vi "方格图标定.vi"() -> ()   [LabVIEW 2018]
uses:
  <vilib>/vision/Calibration.llb/Calibration Reference Points.ctl
  <vilib>/vision/Calibration.llb/Distortion Model.ctl
  <vilib>/vision/Calibration.llb/Distortion Model Types.ctl
  <vilib>/Utility/error.llb/DialogType.ctl
  <vilib>/vision/NI_Vision_Development_Module.lvlib
panel:
  in  "布尔":bool
  out "ROI Descriptor":T1 {"Contours"."Type" items=["No Selection", "Point", "Line", "Rectangle", "Oval", "Polygon", "Freehand Region", "Annulus", "Unused2", "Unused3", "Broken Line", "Freehand Line", "Rotated Rectangle"]}
  in  "生成均值坐标点":bool
  in  "角点增加":bool
  in  "停止按钮":bool
  in  "进行图像标定":bool
  out "标定完成":bool
  out "Location":cluster{"X":sgl, "Y":sgl}
  in  "X轴方向间距":i32
  in  "Y轴方向间距":i32
  in  "Reference Points":T2
  in  "单位选择":u16(ring) items=["Undefined", "Angstr", "Micrometer", "Millimeter", "Centimeter", "Meter", "Kilometer", "Microinch", "Inch", "Feet", "Nautical miles", "Standardmiles", "Steps"]
  out "角点图":T4(plugin-control)
  out "图像尺寸":cluster{"X":u32, "Y":u32}
  in  "删除按钮":bool
  in  "角点检测参数设置":T5={"角点检测算法选择"=0, "Kernel 尺寸"=3, "最小的角点强度"=20.0} {"角点检测算法选择" items=["Harris Corner", "Shi-Tomasi Corner"]; "Kernel 尺寸" min=3 max=7 step=2}
  in  "刷新按钮":bool
  # "方格图标定"
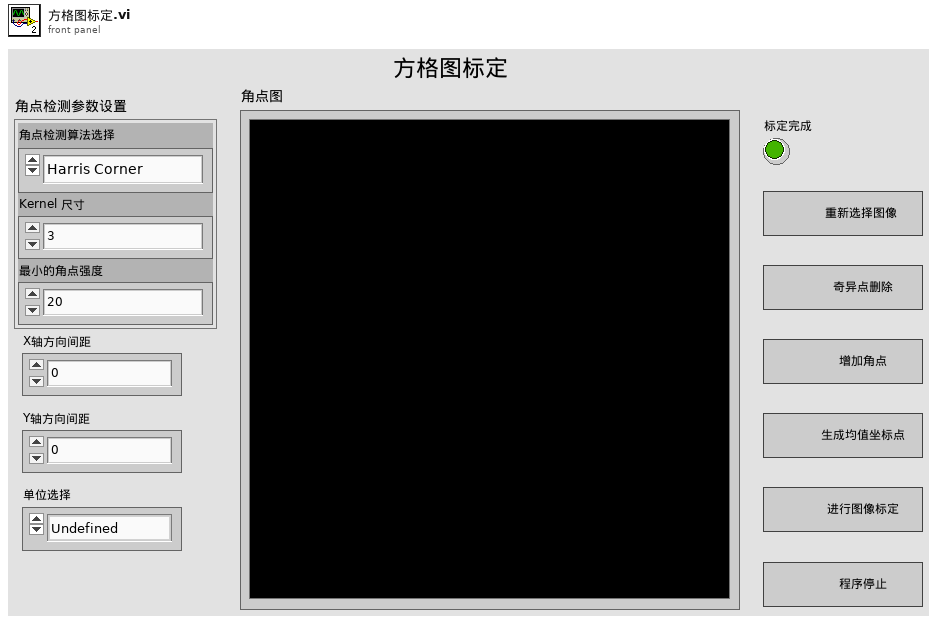
[diagram p1: front panel]
types:
  T1 = typedef "ROI Descriptor" = cluster{"Global Rectangle":i32[], "Contours":cluster{"ID":enum32{"External", "Internal"}, "Type":u32, "Coordinates":i32[]}[]}
  T2 = typedef "Calibration Reference Points.ctl" = cluster{"Pixel Coordinates":cluster{"X":dbl, "Y":dbl}[], "Real World Coordinates":cluster{"X":dbl, "Y":dbl}[], "Unit":T3, "Image Size":cluster{"X":u32, "Y":u32}}
  T3 = typedef "Image Unit" = enum32{"Undefined", "Angström", "Micrometer", "Millimeter", "Centimeter", "Meter", "Kilometer", "Microinch", "Inch", "Feet", "Nautical miles", "Standard miles", "Steps"}
  T4 = typedef "IMAQ Image.ctl" = refnum<image>
  T5 = cluster{"角点检测算法选择":u16, "Kernel 尺寸":i32, "最小的角点强度":dbl}
  T6 = enum8{"Enabled", "Disabled", "Disabled and Grayed Out"}
  T7 = typedef "Image Type" = u32
  T8 = typedef "IMAQ Rectangle" = cluster{"Left":i32, "Top":i32, "Right":i32, "Bottom":i32, "Rotation":dbl}
  T9 = enum32{"Invalid", "Standard", "Closed", "Hidden", "Minimized", "Maximized"}
  T10 = typedef "DialogType.ctl" = u16
  T11 = typedef "Distortion Model.ctl" = cluster{"Distortion Model":T12, "Polynomial Model Setup":cluster{"Radial Coefficient":u32, "Tangential Coefficients ":bool}}
  T12 = typedef "Distortion Model Types.ctl" = i32
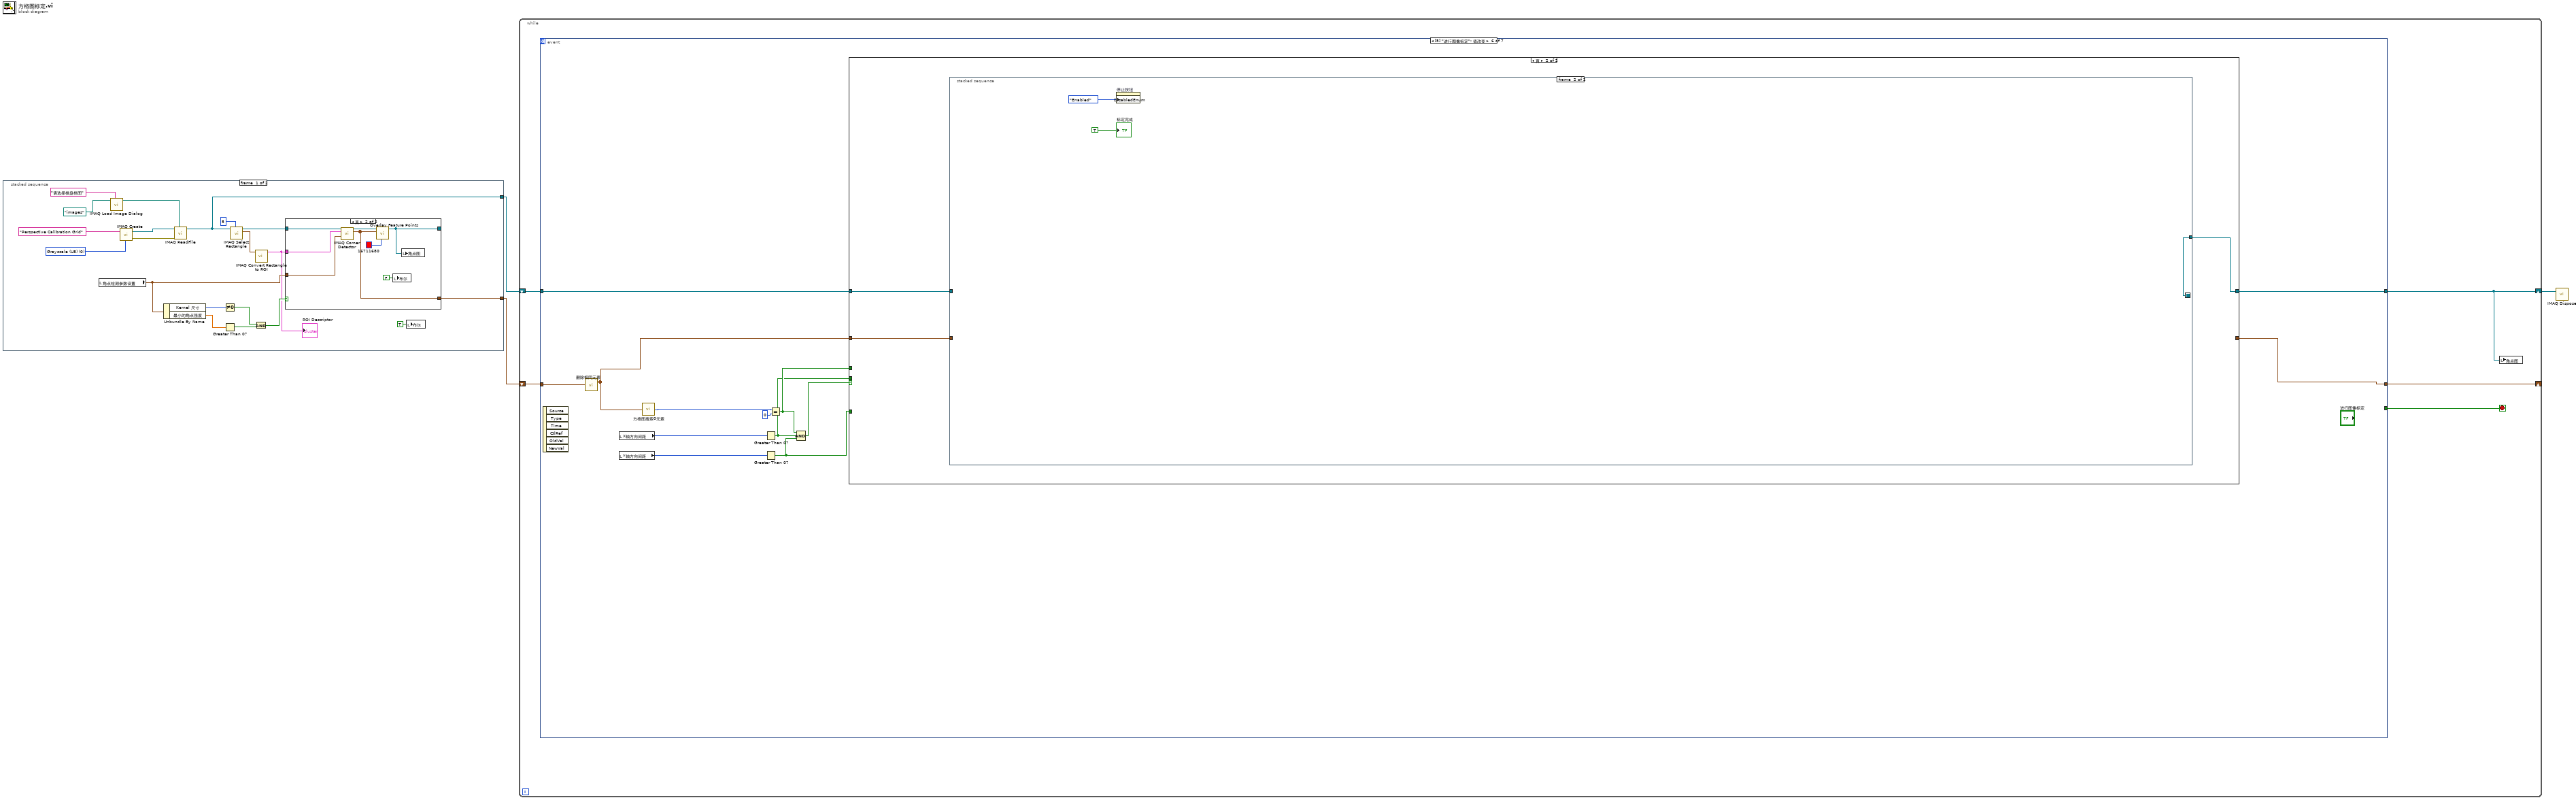
[diagram p0: block diagram]
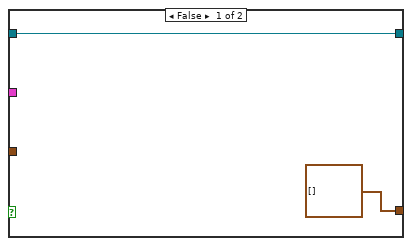
[diagram p2: hidden frame]
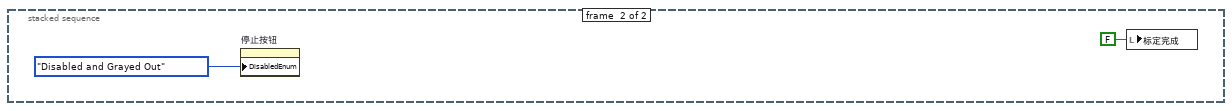
[diagram p3: hidden frame]
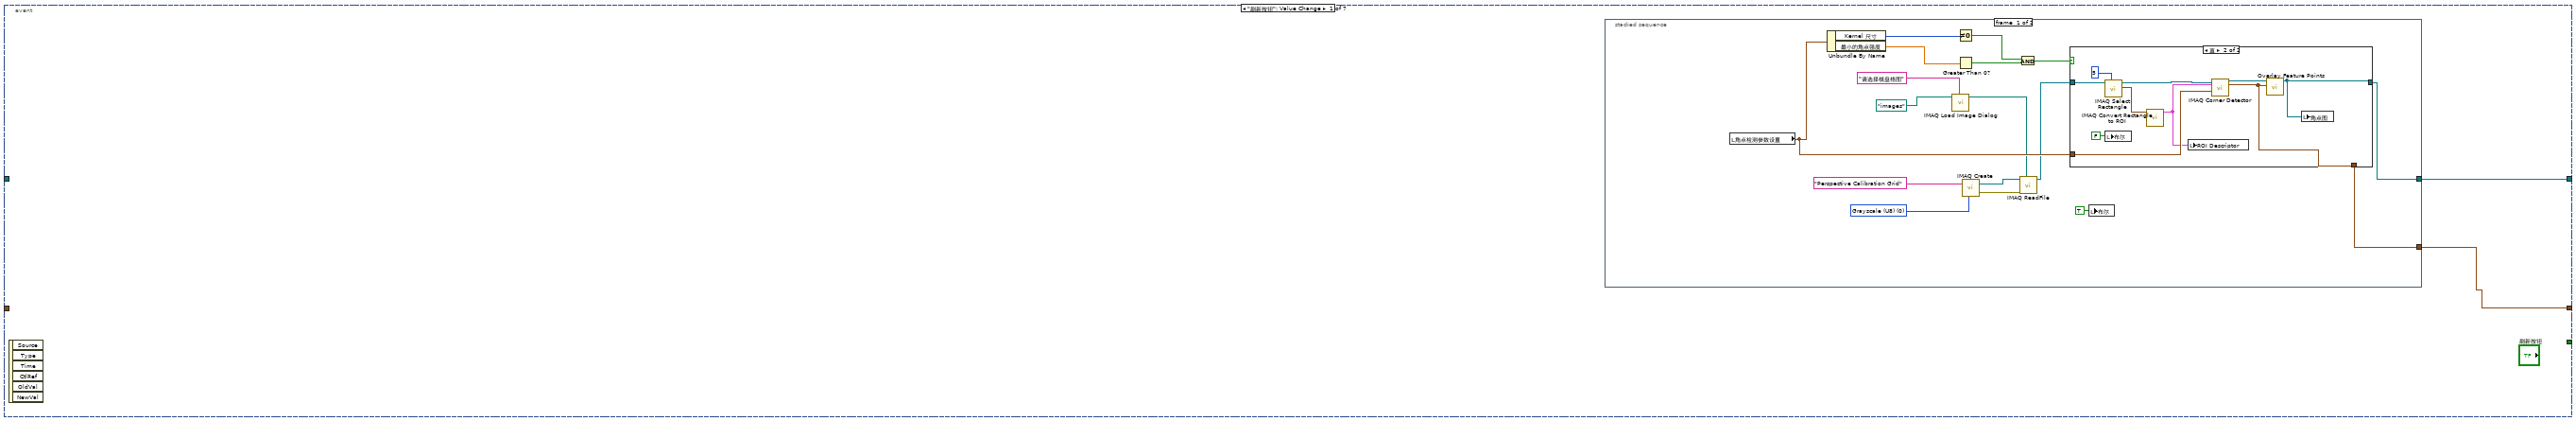
[diagram p4: hidden frame]
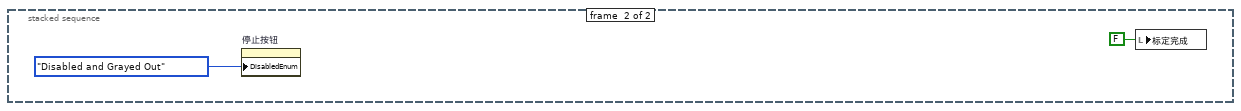
[diagram p6: hidden frame]
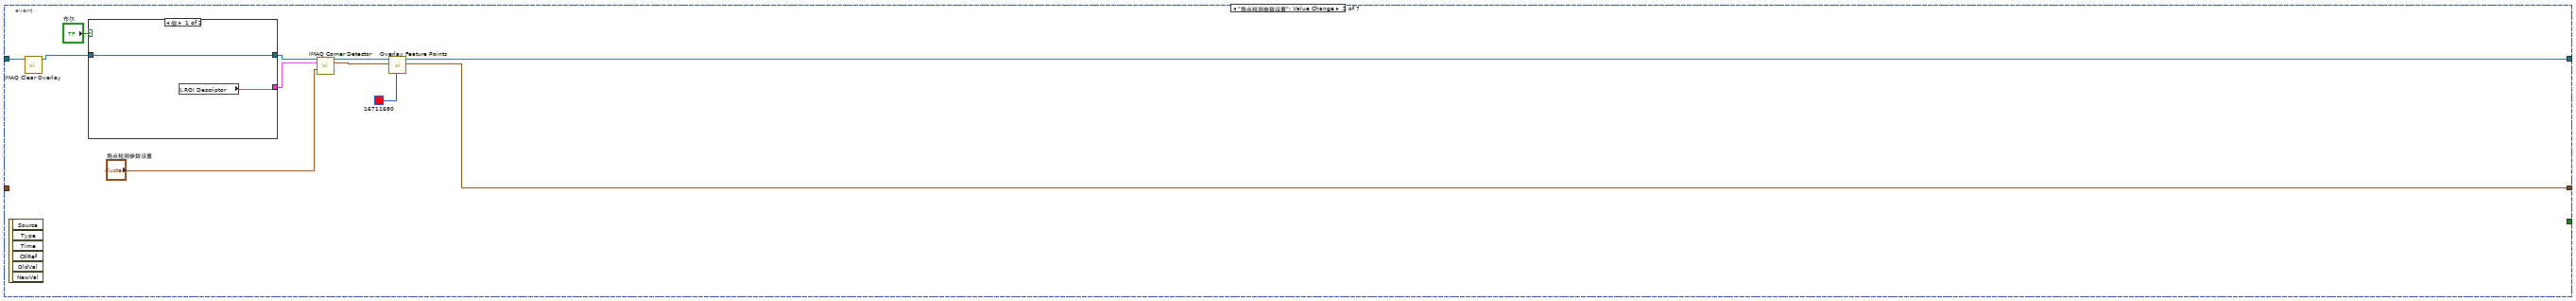
[diagram p7: hidden frame]
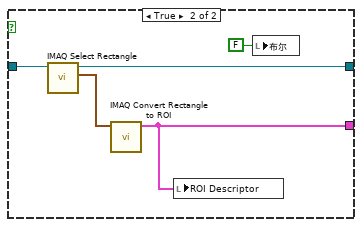
[diagram p8: hidden frame]
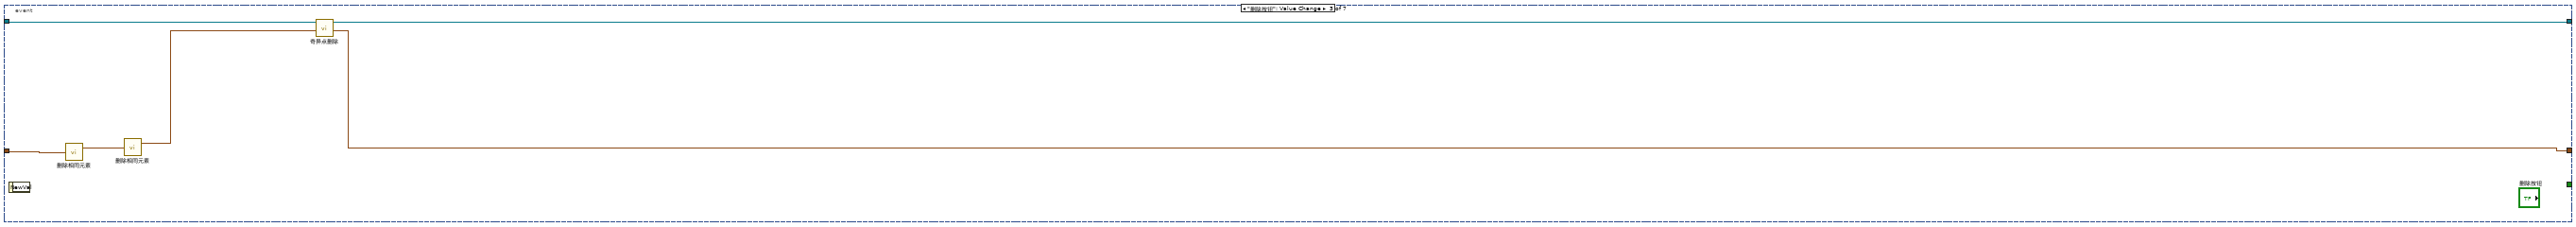
[diagram p9: hidden frame]
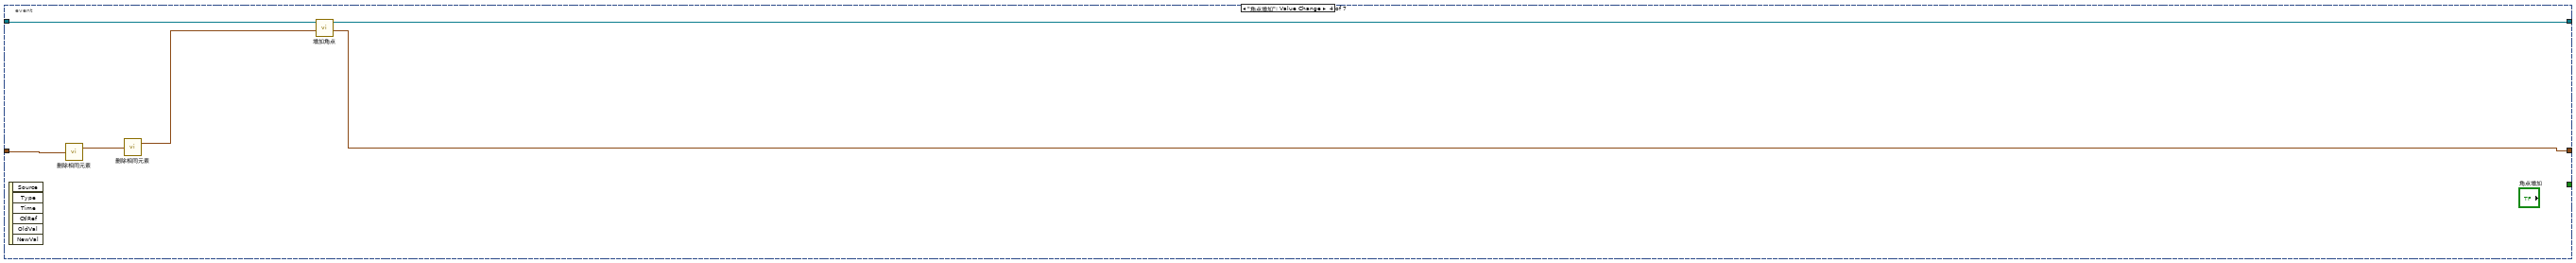
[diagram p10: hidden frame]
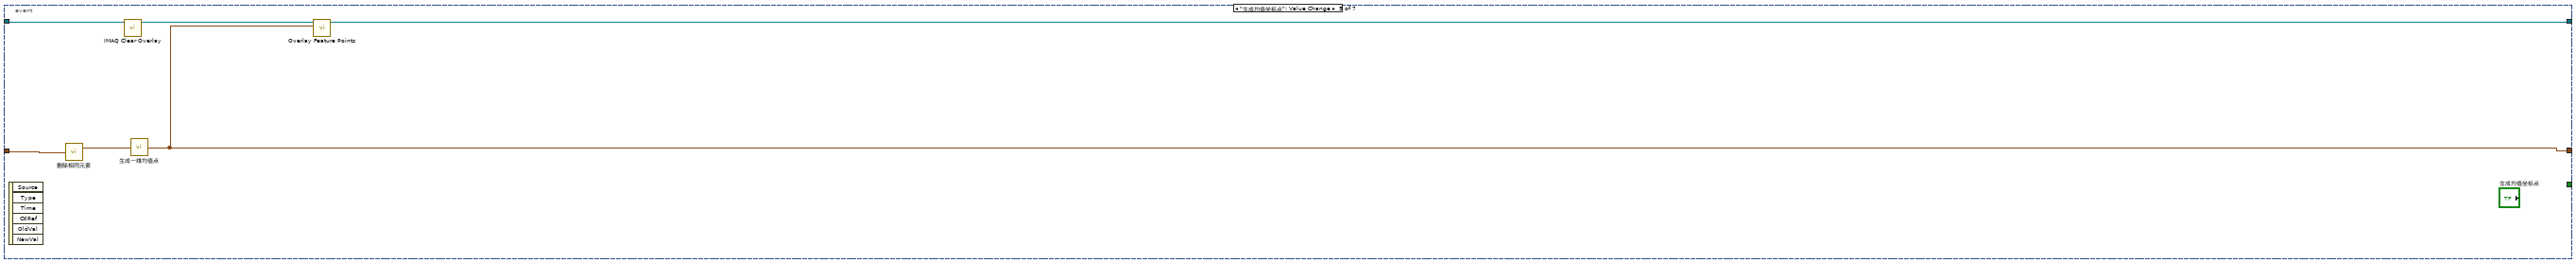
[diagram p11: hidden frame]
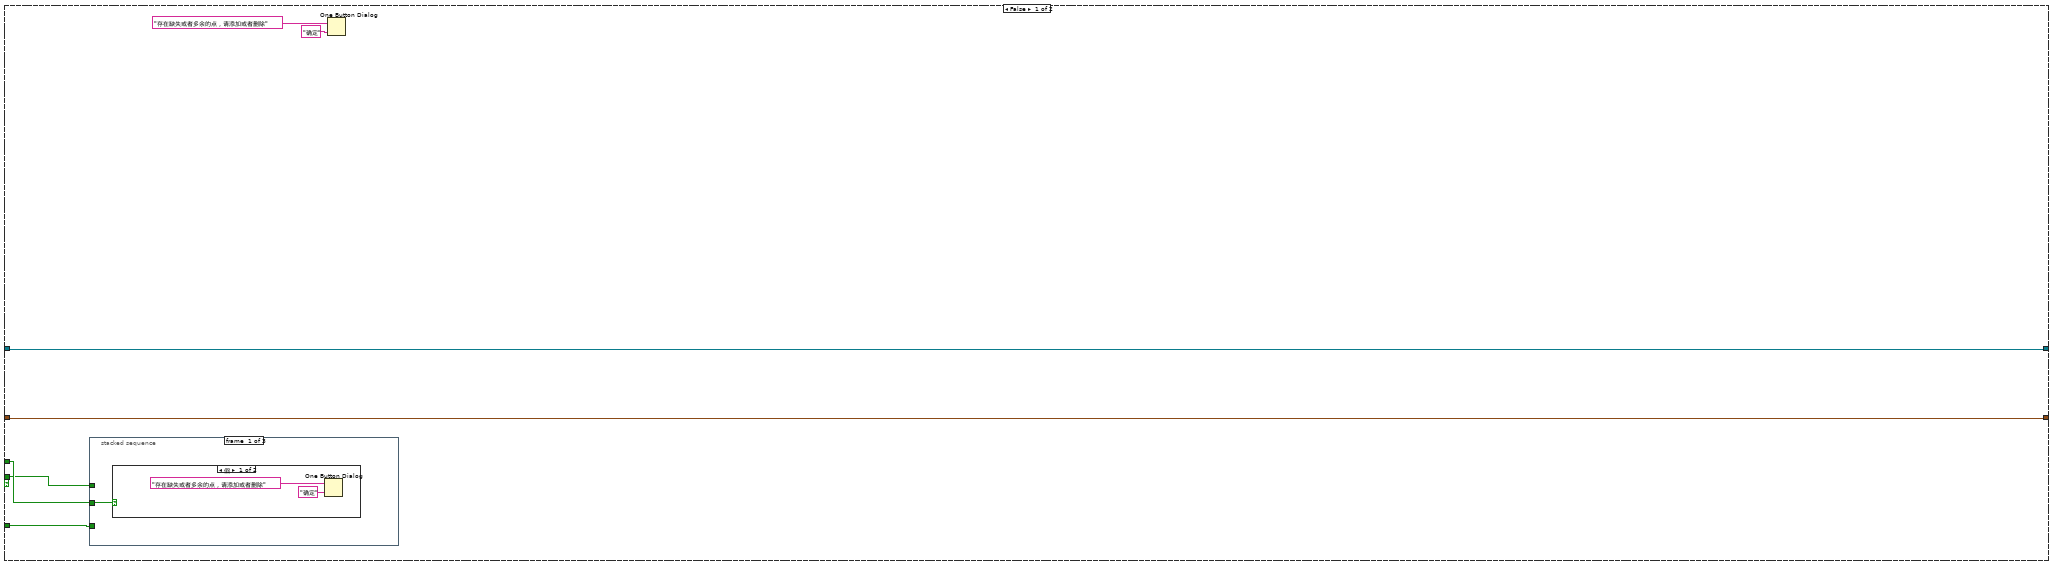
[diagram p12: hidden frame]
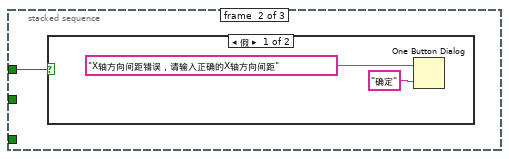
[diagram p14: hidden frame]
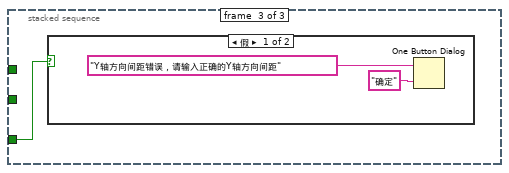
[diagram p16: hidden frame]
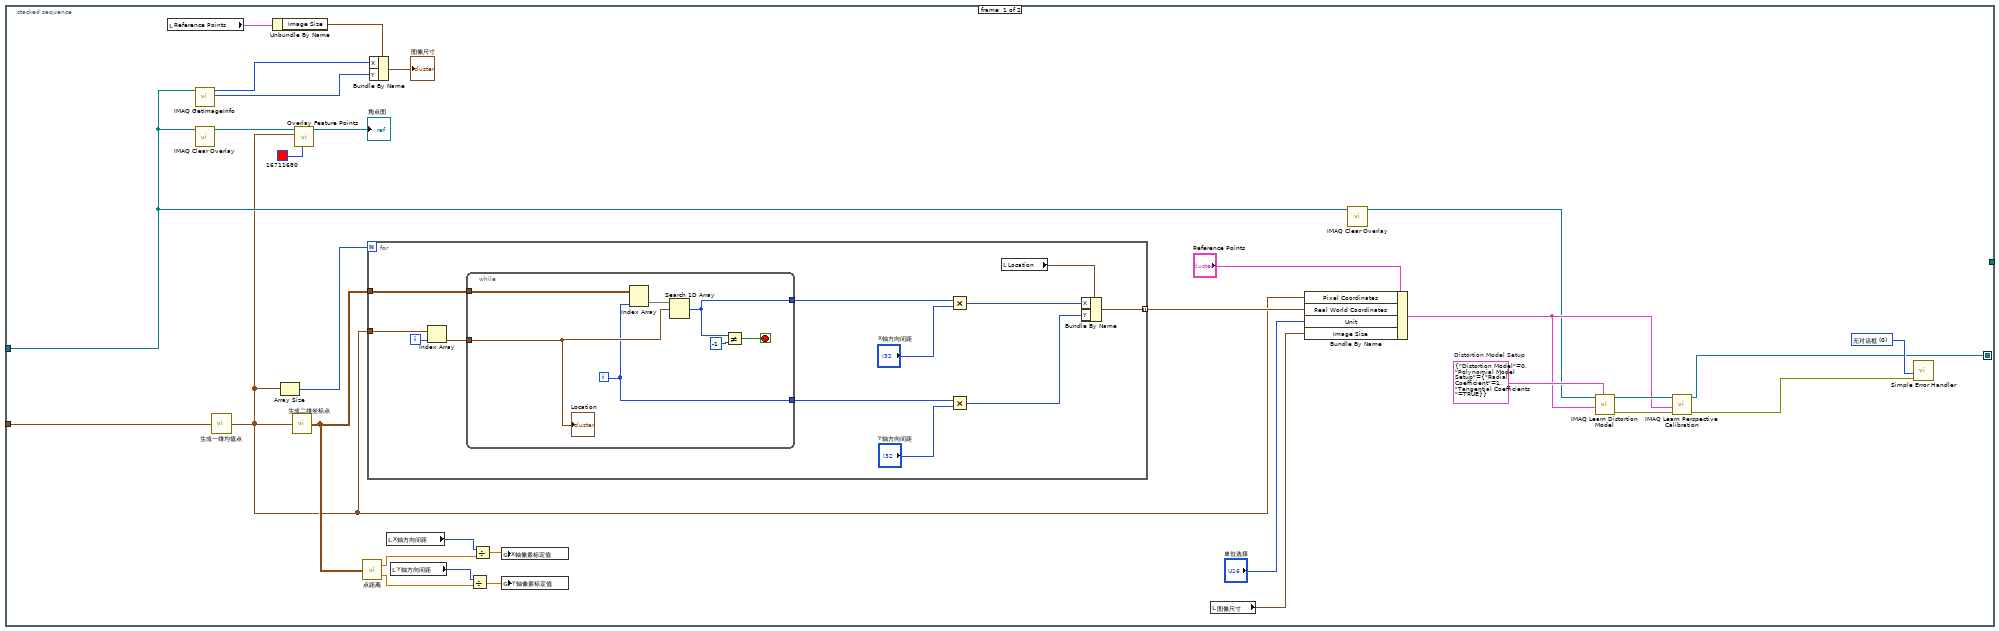
[diagram p18: hidden frame]
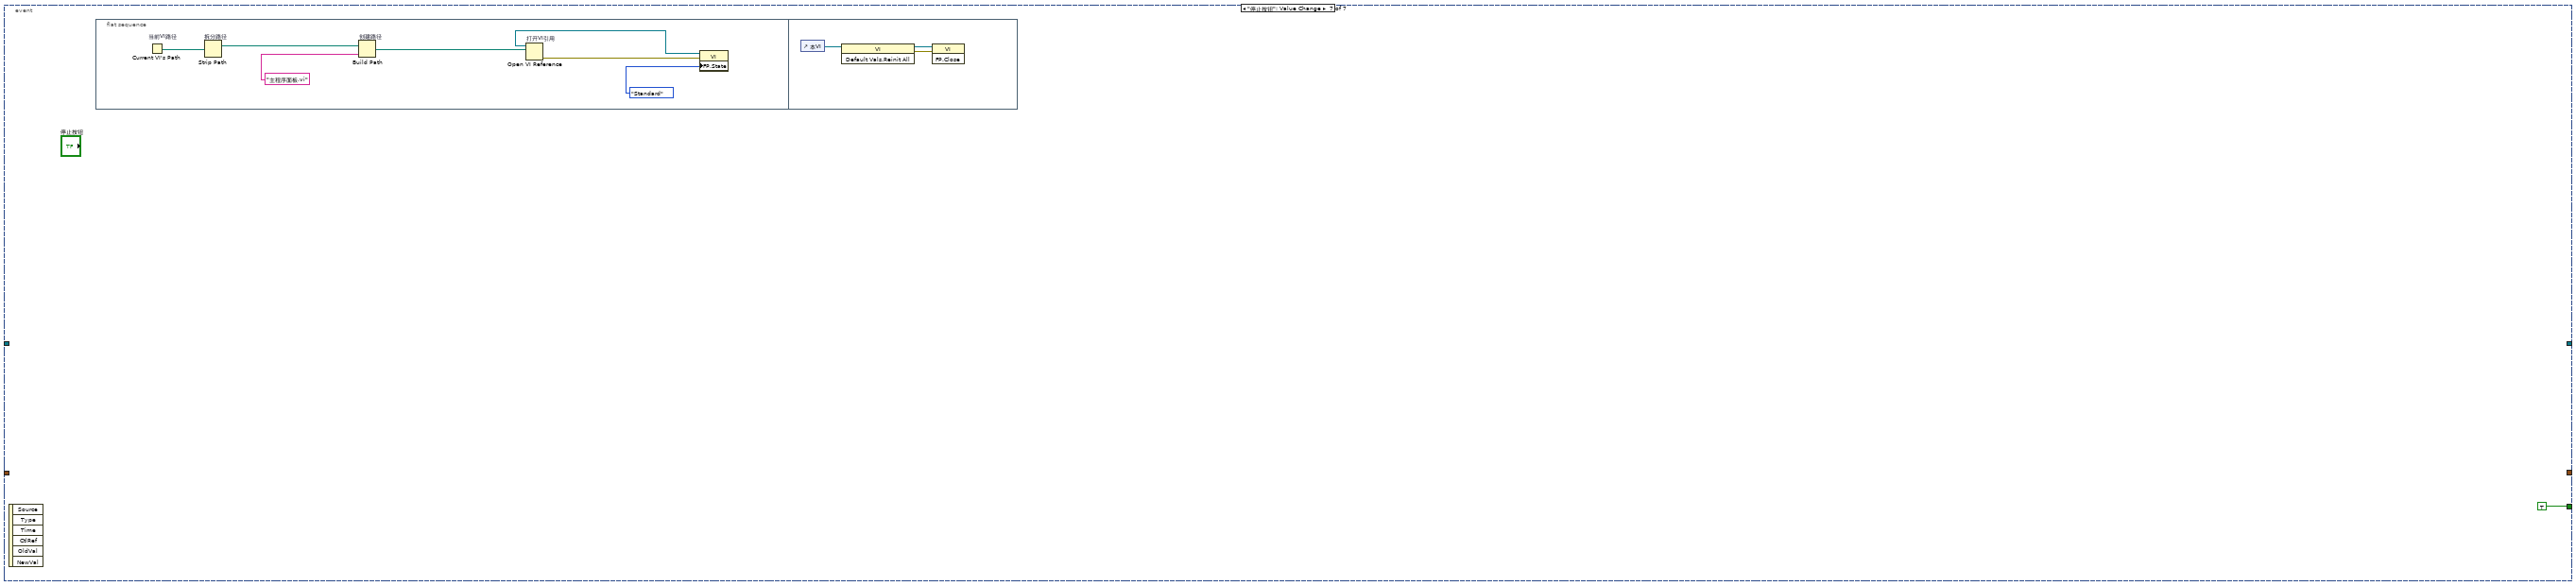
[diagram p19: hidden frame]
diagram:
  n1 = stacked-sequence {
    tunnel: [w10 _] -> w2
    tunnel: [w7 _] -> w1
    frame #0 {
      w11 = T7 0 items=["Grayscale (U8)", "Grayscale (I16)", "Grayscale (SGL)", "Complex (CSG)", "RGB (U32)", "HSL (U32)", "RGB (U64)", "Grayscale (U16)"] ("Image Type")
      n2 = local read "角点检测参数设置"() -> (w18:T5)
      n3 = call "IMAQ Load Image Dialog"("Prompt"="请选择棋盘格图" ("prompt"), "Start Path"=path "images") -> ("Path"=w13:path)  [unwired: 7 in, 2 out]
      n4 = call "IMAQ Create"("Image Name"="Perspective Calibration Grid", "Image Type"=w11) -> ("New Image"=w16:T4, "error out"=w15:errorcluster)  [unwired: 2 in, 1 out]
      n5 = Unbundle By Name(w18) -> ("Kernel 尺寸"=w19:i32, "最小的角点强度"=w20:dbl)
      n6 = call "IMAQ ReadFile"("File Path"=w13, "error in (no error)"=w15, "Image"=w16) -> ("Image Out"=w7:T4)  [unwired: 2 in, 6 out]
      n7 = Not Equal To 0?(x=w19) -> (x != 0?=w21:bool)
      n8 = Greater Than 0?(x=w20) -> (x > 0?=w22:bool)
      n9 = call "IMAQ Select Rectangle"("Window Number (0...15)"=5, "Image In"=w7) -> ("Rectangle"=w9:T8, "Image Out (duplicate)"=w8:T4)  [unwired: 6 in, 2 out]
      n10 = And(x=w21, y=w22) -> (x .and. y?=w23:bool)
      n11 = call "IMAQ Convert Rectangle to ROI"("Rectangle"=w9) -> ("ROI Descriptor"=w5:T1)  [unwired: 8 in, 1 out]
      "ROI Descriptor" <- w5
      n12 = case shown="真" w23 {
        tunnel: w18 -> [_ w33]
        tunnel: [w25 w31] -> _
        tunnel: [cluster{"X":sgl, "Y":sgl}[] [] ("Corner Point Coordinates") w29] -> w10
        tunnel: w5 -> [_ w28]
        tunnel: w8 -> [w25 w27]
        frame False {
        }
        frame True {
          n13 = call "IMAQ Corner Detector"("Image"=w27, "ROI Descriptor"=w28, "Corner Options"=w33) -> ("Image (duplicate)"=w32:T4, "Corner Point Coordinates"=w29:cluster{"X":sgl, "Y":sgl}[])  [unwired: 7 in, 4 out]
          n14 = call "Overlay Feature Points.vi"("Color"=u32 16711680, "Feature Points"=w29, "Image"=w32) -> ("Image Out"=w31:T4)  [unwired: 7 in, 1 out]
          n15 = local write "布尔"(FALSE ("布尔")) -> ()
          n16 = local write "角点图"(w31) -> ()
        }
      }
      n17 = local write "布尔"(TRUE ("布尔")) -> ()
    }
    frame #1 {
      n18 = property on="停止按钮" class="Bool"("DisabledEnum"=T6."Disabled and Grayed Out" ("禁用")) -> ()  [unwired: 2 in, 2 out]
      n19 = local write "标定完成"(FALSE ("标定完成")) -> ()
    }
  }
  n20 = while {
    shift-right: [w36] -> w3
    shift-left: w1 -> [w38]
    shift-right: [w40] -> _
    shift-left: w2 -> [w39]
    stop <- w37 stop-if-true
    n21 = event shown="[5] \"进行图像标定\": 值改变" {
      selector: _ -> [_ _ _ _ _ _ _]
      dyn-events: _ -> [_ _ _ _ _ _ _]
      timeout: _ -> [_ _ _ _ _ _ _]
      tunnel: [w42 w79 w92 w99 w104 w116 _] -> w36
      tunnel: [w41 w77 w94 w98 w105 w117 _] -> w40
      tunnel: w39 -> [_ _ w91 w97 w103 w115 _]
      tunnel: w38 -> [_ w80 w93 w101 w107 w118 _]
      tunnel: [_ _ _ _ _ _ TRUE] -> w37
      event "刷新按钮": Value Change {
        n22 = event-data() -> ()  [unwired: 1 in, 6 out]
        n23 = stacked-sequence {
          tunnel: [w46 _] -> w42
          tunnel: [w45 _] -> w41
          frame #0 {
            w47 = T7 0 items=["Grayscale (U8)", "Grayscale (I16)", "Grayscale (SGL)", "Complex (CSG)", "RGB (U32)", "HSL (U32)", "RGB (U64)", "Grayscale (U16)"] ("Image Type")
            n24 = local read "角点检测参数设置"() -> (w54:T5)
            n25 = Unbundle By Name(w54) -> ("Kernel 尺寸"=w55:i32, "最小的角点强度"=w56:dbl)
            n26 = call "IMAQ Load Image Dialog"("Prompt"="请选择棋盘格图" ("prompt"), "Start Path"=path "images") -> ("Path"=w49:path)  [unwired: 7 in, 2 out]
            n27 = Not Equal To 0?(x=w55) -> (x != 0?=w57:bool)
            n28 = Greater Than 0?(x=w56) -> (x > 0?=w58:bool)
            n29 = call "IMAQ Create"("Image Name"="Perspective Calibration Grid", "Image Type"=w47) -> ("New Image"=w52:T4, "error out"=w51:errorcluster)  [unwired: 2 in, 1 out]
            n30 = And(x=w57, y=w58) -> (x .and. y?=w59:bool)
            n31 = call "IMAQ ReadFile"("File Path"=w49, "error in (no error)"=w51, "Image"=w52) -> ("Image Out"=w44:T4)  [unwired: 2 in, 6 out]
            n32 = case shown="真" w59 {
              tunnel: w54 -> [_ w70]
              tunnel: [w60 w68] -> w46
              tunnel: w44 -> [w60 w66]
              tunnel: [_ w67] -> w45
              frame False {
              }
              frame True {
                n33 = call "IMAQ Select Rectangle"("Window Number (0...15)"=5, "Image In"=w66) -> ("Rectangle"=w64:T8, "Image Out (duplicate)"=w65:T4)  [unwired: 6 in, 2 out]
                n34 = local write "布尔"(FALSE ("布尔")) -> ()
                n35 = call "IMAQ Convert Rectangle to ROI"("Rectangle"=w64) -> ("ROI Descriptor"=w62:T1)  [unwired: 8 in, 1 out]
                n36 = local write "ROI Descriptor"(w62) -> ()
                n37 = call "IMAQ Corner Detector"("Image"=w65, "ROI Descriptor"=w62, "Corner Options"=w70) -> ("Image (duplicate)"=w69:T4, "Corner Point Coordinates"=w67:cluster{"X":sgl, "Y":sgl}[])  [unwired: 7 in, 4 out]
                n38 = call "Overlay Feature Points.vi"("Feature Points"=w67, "Image"=w69) -> ("Image Out"=w68:T4)  [unwired: 8 in, 1 out]
                n39 = local write "角点图"(w68) -> ()
              }
            }
            n40 = local write "布尔"(TRUE ("布尔")) -> ()
          }
          frame #1 {
            n41 = property on="停止按钮" class="Bool"("DisabledEnum"=T6."Disabled and Grayed Out" ("禁用")) -> ()  [unwired: 2 in, 2 out]
            n42 = local write "标定完成"(FALSE ("标定完成")) -> ()
          }
        }
      }
      event "角点检测参数设置": Value Change {
        n43 = event-data() -> ()  [unwired: 1 in, 6 out]
        n44 = call "IMAQ Clear Overlay"("Image"=w80) -> ("Image Out"=w76:T4)  [unwired: 9 in, 1 out]
        n45 = case shown="假" "布尔" {
          tunnel: w76 -> [w83 w89]
          tunnel: [w83 w88] -> w75
          tunnel: [w84 w86] -> w74
          frame False {
            n46 = local read "ROI Descriptor"() -> (w84:T1)
          }
          frame True {
            n47 = call "IMAQ Select Rectangle"("Image In"=w89) -> ("Rectangle"=w87:T8, "Image Out (duplicate)"=w88:T4)  [unwired: 7 in, 2 out]
            n48 = call "IMAQ Convert Rectangle to ROI"("Rectangle"=w87) -> ("ROI Descriptor"=w86:T1)  [unwired: 8 in, 1 out]
            n49 = local write "ROI Descriptor"(w86) -> ()
            n50 = local write "布尔"(FALSE ("布尔")) -> ()
          }
        }
        n51 = call "IMAQ Corner Detector"("Image"=w75, "ROI Descriptor"=w74, "Corner Options"="角点检测参数设置") -> ("Image (duplicate)"=w78:T4, "Corner Point Coordinates"=w77:cluster{"X":sgl, "Y":sgl}[])  [unwired: 7 in, 4 out]
        n52 = call "Overlay Feature Points.vi"("Color"=u32 16711680, "Feature Points"=w77, "Image"=w78) -> ("Image Out"=w79:T4)  [unwired: 7 in, 1 out]
      }
      event "删除按钮": Value Change {
        n53 = event-data() -> ()  [unwired: 1 in, 1 out]
        n54 = call "删除相同元素.vi"("输入"=w91) -> ("输出"=w90:cluster{"X":sgl, "Y":sgl}[])  [unwired: 1 out]
        n55 = call "删除相同元素.vi"("输入"=w90) -> ("输出"=w95:cluster{"X":sgl, "Y":sgl}[])  [unwired: 1 out]
        n56 = call "奇异点删除.vi"("原始角点坐标"=w95, "Image In"=w93) -> ("原始角点坐标 2"=w94:cluster{"X":sgl, "Y":sgl}[], "角点图"=w92:T4)  [unwired: 6 in]
      }
      event "角点增加": Value Change {
        n57 = event-data() -> ()  [unwired: 1 in, 6 out]
        n58 = call "删除相同元素.vi"("输入"=w97) -> ("输出"=w96:cluster{"X":sgl, "Y":sgl}[])  [unwired: 1 out]
        n59 = call "删除相同元素.vi"("输入"=w96) -> ("输出"=w100:cluster{"X":sgl, "Y":sgl}[])  [unwired: 1 out]
        n60 = call "增加角点.vi"("原始角点坐标"=w100, "Image In"=w101) -> ("原始角点坐标 2"=w98:cluster{"X":sgl, "Y":sgl}[], "角点图"=w99:T4)  [unwired: 8 in]
      }
      event "生成均值坐标点": Value Change {
        n61 = event-data() -> ()  [unwired: 1 in, 6 out]
        n62 = call "删除相同元素.vi"("输入"=w103) -> ("输出"=w102:cluster{"X":sgl, "Y":sgl}[])  [unwired: 1 out]
        n63 = call "IMAQ Clear Overlay"("Image"=w107) -> ("Image Out"=w106:T4)  [unwired: 9 in, 1 out]
        n64 = call "生成一维均值点.vi"("无序一维坐标点"=w102) -> ("无序一维均值坐标点"=w105:cluster{"X":sgl, "Y":sgl}[])
        n65 = call "Overlay Feature Points.vi"("Feature Points"=w105, "Image"=w106) -> ("Image Out"=w104:T4)  [unwired: 8 in, 1 out]
      }
      event "进行图像标定": Value Change {
        n66 = event-data() -> ()  [unwired: 1 in, 6 out]
        n67 = call "删除相同元素.vi"("输入"=w115) -> ("输出"=w114:cluster{"X":sgl, "Y":sgl}[])  [unwired: 1 out]
        n68 = local read "X轴方向间距"() -> (w113:i32)
        n69 = local read "Y轴方向间距"() -> (w112:i32)
        n70 = call "方格图搜索0元素.vi"("无序一维坐标点"=w114) -> ("数值输入控件"=w119:i32)
        n71 = Greater Than 0?(x=w113) -> (x > 0?=w109:bool)
        n72 = Greater Than 0?(x=w112) -> (x > 0?=w108:bool)
        n73 = Equal?(x=w119, y=0) -> (x = y?=w110:bool)
        n74 = Compound Arithmetic op=AND(w110, w109, w108) -> (w111:bool)
        n75 = case shown="真" w111 {
          tunnel: w114 -> [w125 w139]
          tunnel: w118 -> [w124 w138]
          tunnel: [w125 _] -> w117
          tunnel: [w124 w137] -> w116
          tunnel: w110 -> [w123 _]
          tunnel: w109 -> [w122 _]
          tunnel: w108 -> [w121 _]
          frame False {
            n76 = stacked-sequence {
              tunnel: w123 -> [w128 _ _]
              tunnel: w122 -> [_ w131 _]
              tunnel: w121 -> [_ _ w134]
              frame #0 {
                n77 = case shown="假" w128 {
                  frame False {
                    n78 = One Button Dialog(message="存在缺失或者多余的点，请添加或者删除" ("消息"), button name ("OK")="确定" ("按钮名称（“确定”）")) -> ()  [unwired: 1 out]
                  }
                  frame True {
                  }
                }
              }
              frame #1 {
                n79 = case shown="假" w131 {
                  frame False {
                    n80 = One Button Dialog(message="X轴方向间距错误，请输入正确的X轴方向间距" ("消息"), button name ("OK")="确定" ("按钮名称（“确定”）")) -> ()  [unwired: 1 out]
                  }
                  frame True {
                  }
                }
              }
              frame #2 {
                n81 = case shown="假" w134 {
                  frame False {
                    n82 = One Button Dialog(message="Y轴方向间距错误，请输入正确的Y轴方向间距" ("消息"), button name ("OK")="确定" ("按钮名称（“确定”）")) -> ()  [unwired: 1 out]
                  }
                  frame True {
                  }
                }
              }
            }
            n83 = One Button Dialog(message="存在缺失或者多余的点，请添加或者删除" ("消息"), button name ("OK")="确定" ("按钮名称（“确定”）")) -> ()  [unwired: 1 out]
          }
          frame True {
            n84 = stacked-sequence {
              seq-local: [w140 _] -> [_ w192]
              tunnel: w139 -> [w157 _]
              tunnel: w138 -> [w152 _]
              tunnel: [_ w192] -> w137
              frame #0 {
                w166 = T10 0 items=["无对话框", "确定信息", "继续或停止信息", "确定信息＋警告", "继续/停止+警告"] ("type of dialog (OK msg:1)")
                w168 = T11 {"Distortion Model"=0, "Polynomial Model Setup"={"Radial Coefficient"=1, "Tangential Coefficients "=TRUE}}  # Distortion Model Setup
                n85 = local read "Reference Points"() -> (w155:T2)
                n86 = call "IMAQ GetImageInfo"("Image"=w152) -> ("Y Resolution"=w151:i32, "X Resolution"=w156:i32)  [unwired: 3 in, 6 out]
                n87 = call "IMAQ Clear Overlay"("Image"=w152) -> ("Image Out"=w160:T4)  [unwired: 9 in, 1 out]
                n88 = call "生成一维均值点.vi"("无序一维坐标点"=w157) -> ("无序一维均值坐标点"=w142:cluster{"X":sgl, "Y":sgl}[])
                n89 = Unbundle By Name(w155) -> ("Image Size"=w154:cluster{"X":u32, "Y":u32})
                n90 = Array Size(array=w142) -> (size(s)=w170:i32)
                n91 = call "生成二维坐标点.vi"("输入无序一维坐标点"=w142) -> ("输出有序二维坐标点"=w149:cluster{"X":sgl, "Y":sgl}[][])
                n92 = call "Overlay Feature Points.vi"("Color"=u32 16711680, "Feature Points"=w142, "Image"=w160) -> ("Image Out"=→"角点图":T4)  [unwired: 7 in, 1 out]
                n93 = call "点距离.vi"("二维点阵"=w149) -> ("X间距"=w147:sgl, "Y间距"=w145:sgl)
                n94 = for {
                  N: w170 -> [_]
                  tunnel: w149 -> [w181]
                  tunnel: w142 -> [w171]
                  tunnel: [w172] -> w150 mode=indexing
                  i -> [w182]
                  n95 = Index Array(array=w171, index=w182) -> (element=w180:cluster{"X":sgl, "Y":sgl})
                  n96 = while {
                    tunnel: w181 -> [w188]
                    tunnel: w180 -> [w189]
                    tunnel: [w184] -> w176
                    tunnel: [w185] -> w177
                    i -> [w184]
                    stop <- w186 stop-if-true
                    n97 = Index Array(array=w188, index (col)=w184) -> (element=w183:cluster{"X":sgl, "Y":sgl}[])  [unwired: 1 in]
                    n98 = Search 1D Array(1D array=w183, element=w189) -> (index of element=w185:i32)  [unwired: 1 in]
                    n99 = Not Equal?(x=w185, y=-1) -> (x != y?=w186:bool)
                    "Location" <- w189
                  }
                  n100 = Multiply(x=w177, y="X轴方向间距") -> (x*y=w175:i32)
                  n101 = Multiply(x=w176, y="Y轴方向间距") -> (x*y=w174:i32)
                  n102 = local read "Location"() -> (w173:cluster{"X":sgl, "Y":sgl})
                  n103 = Bundle By Name(cluster=w173, "X"=w175, "Y"=w174) -> (w172:cluster{"X":sgl, "Y":sgl})
                }
                n104 = Bundle By Name(cluster=w154, "X"=w156, "Y"=w151) -> (→"图像尺寸":cluster{"X":u32, "Y":u32})
                n105 = local read "X轴方向间距"() -> (w148:i32)
                n106 = local read "Y轴方向间距"() -> (w146:i32)
                n107 = Divide(x=w146, y=w145) -> (x/y=w143:sgl)
                n108 = Divide(x=w148, y=w147) -> (x/y=w144:sgl)
                n109 = global write "全局变量.vi" "X轴像素标定值"(w144) -> ()
                n110 = global write "全局变量.vi" "Y轴像素标定值"(w143) -> ()
                n111 = local read "图像尺寸"() -> (w162:cluster{"X":u32, "Y":u32})
                n112 = Bundle By Name(cluster="Reference Points", "Pixel Coordinates"=w142, "Real World Coordinates"=w150, "Unit"="单位选择", "Image Size"=w162) -> (w164:T2)
                n113 = call "IMAQ Clear Overlay"("Image"=w152) -> ("Image Out"=w161:T4)  [unwired: 9 in, 1 out]
                n114 = call "IMAQ Learn Distortion Model"("Distortion Model Setup"=w168, "Reference Points"=w164, "Calibration Template Image"=w161) -> ("error out"=w167:errorcluster, "Calibration Template Image Out"=w169:T4)  [unwired: 3 in, 4 out]
                n115 = call "IMAQ Learn Perspective Calibration"("error in (no error)"=w167, "Reference Points"=w164, "Calibration Template Image"=w169) -> ("error out"=w141:errorcluster, "Calibration Template Image Out"=w140:T4)  [unwired: 1 in, 6 out]
                n116 = call <vilib>:"Simple Error Handler.vi"("type of dialog (OK msg:1)"=w166, "error in (no error)"=w141) -> ()  [unwired: 3 in, 5 out]
              }
              frame #1 {
                n117 = property on="停止按钮" class="Bool"("DisabledEnum"=T6."Enabled" ("禁用")) -> ()  [unwired: 2 in, 2 out]
                "标定完成" <- TRUE ("标定完成")
              }
            }
          }
        }
      }
      event "停止按钮": Value Change {
        n118 = event-data() -> ()  [unwired: 1 in, 6 out]
        n119 = flat-sequence {
          frame #0 {
            n120 = Current VI's Path "当前VI路径"() -> (path=w198:path)
            n121 = Strip Path "拆分路径"(path=w198) -> (stripped path=w200:path)  [unwired: 1 out]
            n122 = Build Path "创建路径"(base path=w200, name or relative path="主程序面板.vi" ("名称或相对路径")) -> (appended path=w199:path)
            n123 = Open VI Reference "打开VI引用"(vi path=w199) -> (vi reference=w197:refnum<vi>, error out=w196:errorcluster)  [unwired: 5 in]
            n124 = property class="VI"(reference=w197, error in=w196, "FP.State"=T9."Standard" ("前面板窗口:状态")) -> ()  [unwired: 2 out]
          }
          frame #1 {
            n125 = control-ref of="本VI"() -> (w201:refnum<vi>)
            n126 = invoke class="VI" method="Default Vals.Reinit All"(reference=w201) -> (reference out=w202:refnum<vi>, error out=w203:errorcluster)  [unwired: 2 in, 1 out]
            n127 = invoke class="VI" method="FP.Close"(reference=w202, error in=w203) -> ()  [unwired: 1 in, 3 out]
          }
        }
      }
    }
    n128 = local write "角点图"(w36) -> ()
  }
  n129 = call "IMAQ Dispose"("Image"=w3) -> ()  [unwired: 5 in, 1 out]
